vi "DrawCells.vi"(8 "error in (no error)":errorcluster, 10 "Cell Size":i32, 11 "Sudoku.lvclass in":refnum<class "Sudoku.lvclass">) -> (0 "error out":errorcluster, 3 "Sudoku.lvclass out":refnum<class "Sudoku.lvclass">)   [LabVIEW 2021, in "Sudoku.lvclass"]
uses:
  Sudoku.lvclass
  Sudoku.lvclass/Sudoku.ctl
  Cell/Cell.lvclass
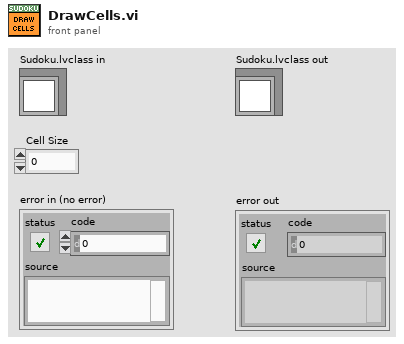
[diagram p1: front panel]
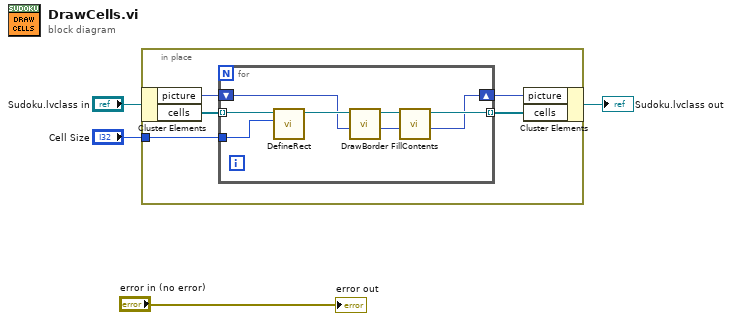
[diagram p0: block diagram]
diagram:
  n1 = in-place {
    in-place-border: "Cell Size" -> [w6]
    n2 = in-place-cluster #1("Sudoku.lvclass in") -> ("picture"=w9:picture, "cells"=w7:refnum<class "Cell.lvclass">[])
    n3 = for {
      shift-right: [w10] -> w8
      shift-left: w9 -> [w14]
      tunnel: w7 -> [w17] mode=indexing
      tunnel: w6 -> [w15]
      tunnel: [w12] -> w5 mode=indexing
      n4 = call "DefineRect.vi"("cell size"=w15, "Cell in"=w17) -> ("Cell out"=w16:refnum<class "Cell.lvclass">)  [unwired: 9 in]
      n5 = call "DrawBorder.vi"("display in"=w14, "Cell in"=w16) -> ("display out"=w11:picture, "Cell out"=w13:refnum<class "Cell.lvclass">)  [unwired: 8 in]
      n6 = call "FillContents.vi"("display in"=w11, "Cell in"=w13) -> ("display out"=w10:picture, "Cell out"=w12:refnum<class "Cell.lvclass">)  [unwired: 8 in]
    }
    n7 = in-place-cluster #1("picture"=w8, "cells"=w5) -> (→"Sudoku.lvclass out":refnum<class "Sudoku.lvclass">)
  }
  "error out" <- "error in (no error)"
